vi "newTestCheck.vi"() -> (1 "设备编号 2":string, 2 "测试方式 2":enum32{"手动测试", "自动测试"}(ring), 3 "测试类型 2":enum32{"INC", "MOP"}(ring))   [LabVIEW 2017]
panel:
  in  "取消按钮":bool
  in  "确定按钮":bool
  in  "测试类型":enum32{"INC", "MOP"}(radio)
  in  "设备编号":string
  in  "测试方式":enum32{"手动测试", "自动测试"}(radio)
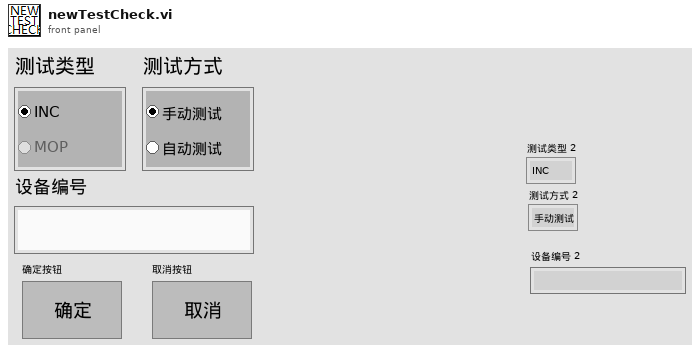
[diagram p1: front panel]
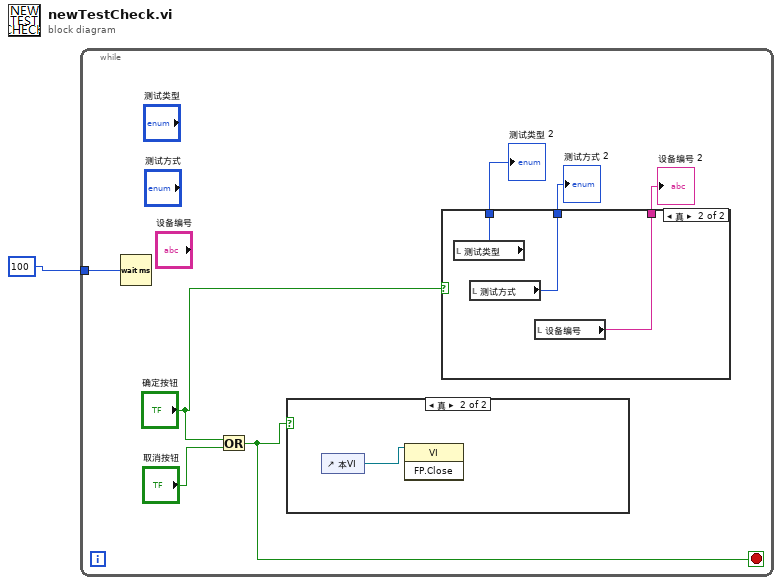
[diagram p0: block diagram]
diagram:
  n1 = while {
    tunnel: 100 -> [w7]
    stop <- w8 stop-if-true
    n2 = Wait (ms)(milliseconds to wait=w7) -> ()  [unwired: 1 out]
    n3 = Or(x="确定按钮", y="取消按钮") -> (x .or. y?=w8:bool)
    n4 = case shown="真" w8 {
      frame False {
      }
      frame True {
        n5 = control-ref of="本VI"() -> (w12:refnum<vi>)
        n6 = invoke class="VI" method="FP.Close"(reference=w12) -> ()  [unwired: 2 in, 3 out]
      }
    }
    n7 = case shown="真" "确定按钮" {
      tunnel: [_ w11] -> w5
      tunnel: [_ w10] -> w4
      tunnel: [_ w9] -> w3
      frame False {
      }
      frame True {
        n8 = local read "测试类型"() -> (w11:enum32{"INC", "MOP"})
        n9 = local read "测试方式"() -> (w10:enum32{"手动测试", "自动测试"})
        n10 = local read "设备编号"() -> (w9:string)
      }
    }
    "测试类型 2" <- w5
    "测试方式 2" <- w4
    "设备编号 2" <- w3
  }
